vi "selectTimer.vi"(8 "error in (no error)":errorcluster, 10 "timer":sgl=0.001 min=0.001 max=1000000, 11 "Electrometer in":refnum<class "Electrometer.lvclass">) -> (0 "error out":errorcluster, 3 "Electrometer out":refnum<class "Electrometer.lvclass">)   [LabVIEW 2016, in "Electrometer.lvclass"]
uses:
  Electrometer.lvclass
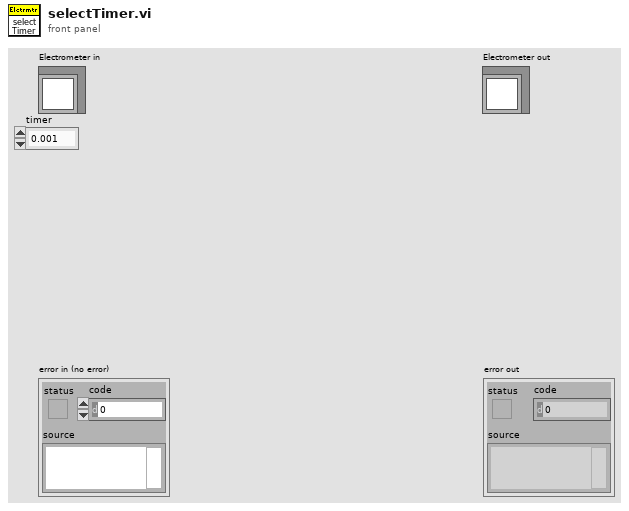
[diagram p1: front panel]
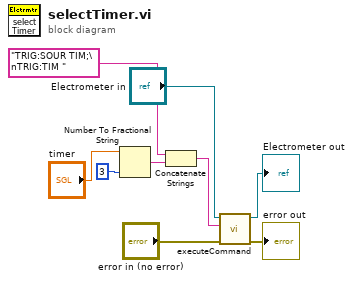
[diagram p0: block diagram]
diagram:
  n1 = Number To Fractional String(number="timer", precision (6)=i16 3) -> (F-format string=w4:string)  [unwired: 2 in]
  n2 = Concatenate Strings("TRIG:SOUR TIM;\nTRIG:TIM " ("command"), w4) -> (w2:string)
  n3 = call "executeCommand.vi"("error in (no error)"="error in (no error)", "command"=w2, "Electrometer in"="Electrometer in") -> ("error out"=→"error out":errorcluster, "Electrometer out"=→"Electrometer out":refnum<class "Electrometer.lvclass">)  [unwired: 7 in]
